vi "split hierarchy.vi"(8 "error in":errorcluster, 10 "UID to split":string, 11 "hierarchy structure":T1) -> (0 "error out":errorcluster, 1 "UIDs moved":string[](array[string]), 2 "hierarchy containing UID":T1, 3 "hierarchy excluding UID":T1)   [LabVIEW 2023, in "CEF.lvlib"]
doc: "Splits a hierarchy at a given instance ID. The first output contains the original tree without the instance specified or any of its children. The second output contains the specified instance and all children, with the specified instance as the new root.Copyright 2017 National Instruments Corporation\n\nLicensed under the Apache License, Version 2.0 (the \"License\"); you may not use this file except in compliance with the License. You may obtain a copy of the License at http://www.apache.org/licenses/LICENSE-2.0\nUnless required by applicable law or agreed to in writing, software distributed under the License is distributed on an \"AS IS\" BASIS, WITHOUT WARRANTIES OR CONDITIONS OF ANY KIND, either express or implied. See the License for the specific language governing permissions and limitations under the License."
uses:
  CEF.lvlib
  hierarchy element.ctl
  hierarchy repo/full hierarchy.ctl
  hierarchy repo/CEF_HierarchyRepo.lvclass
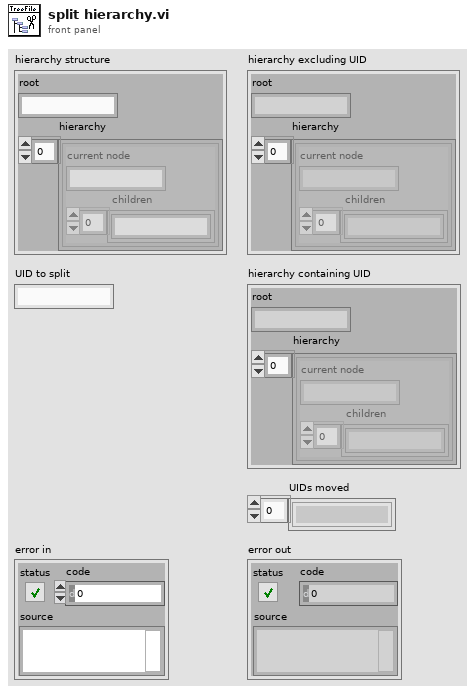
[diagram p1: front panel]
types:
  T1 = typedef "CEF.lvlib/CEF_HierarchyRepo.lvclass/full hierarchy.ctl" = cluster{"root":string, "hierarchy":T2[]}
  T2 = typedef "CEF.lvlib/hierarchy element.ctl" = cluster{"current node":string, "children":string[]}
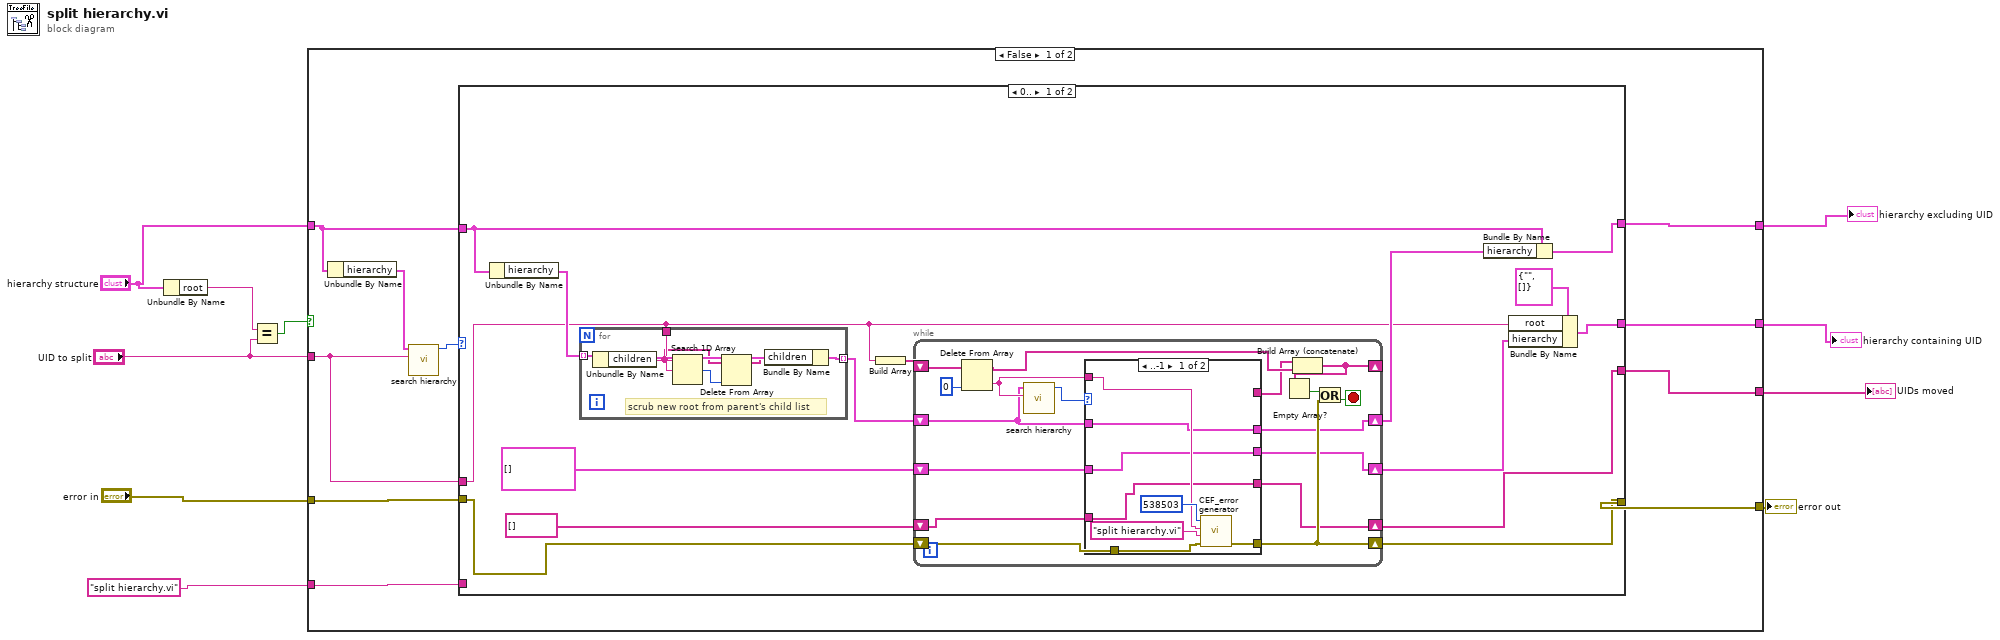
[diagram p0: block diagram]
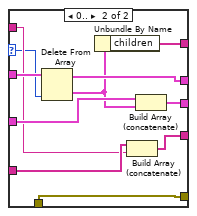
[diagram p2: hidden frame]
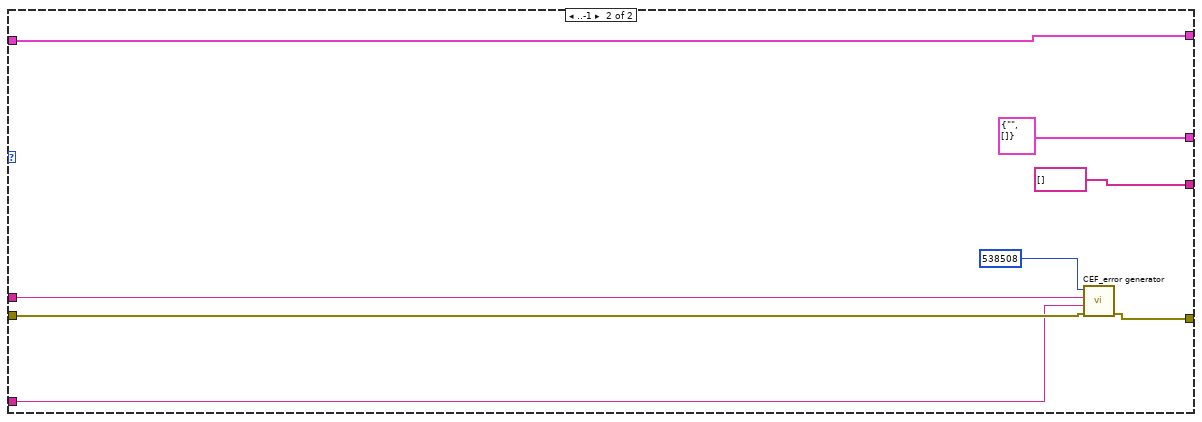
[diagram p3: hidden frame]
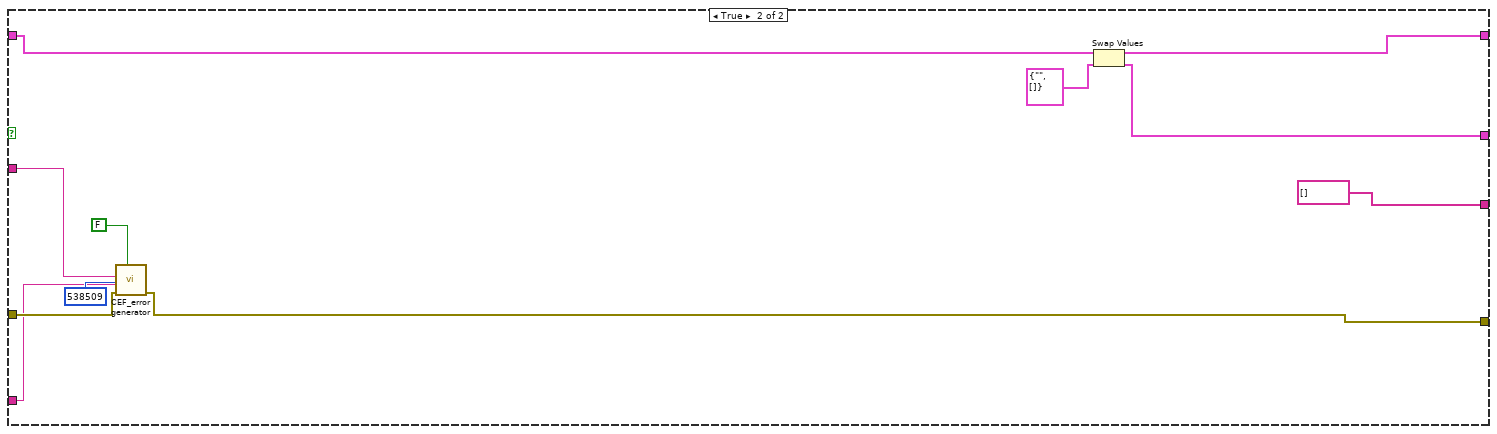
[diagram p4: hidden frame]
diagram:
  n1 = Unbundle By Name("hierarchy structure") -> ("root"=w8:string)
  n2 = Equal?(x=w8, y="UID to split") -> (x = y?=w6:bool)
  n3 = case shown="False" w6 {
    tunnel: "error in" -> [w20 w95]
    tunnel: [w18 w94] -> w9
    tunnel: "UID to split" -> [w17 w93]
    tunnel: [w14 w88] -> w5
    tunnel: "hierarchy structure" -> [w13 w89]
    tunnel: [w11 w86] -> w3
    tunnel: "split hierarchy.vi" ("source") -> [w16 w91]
    tunnel: [w12 string[] [] ("UIDs moved")] -> w1
    frame False {
      n4 = Unbundle By Name(w13) -> ("hierarchy"=w15:T2[])
      n5 = call "search hierarchy.vi"("ID"=w17, "hierarchy"=w15) -> ("index"=w19:i32)  [unwired: 9 in]
      n6 = case shown="0.." w19 {
        tunnel: w20 -> [w25 w84]
        tunnel: [w24 w83] -> w18
        tunnel: w17 -> [w21 w82]
        tunnel: w16 -> [_ w81]
        tunnel: [w33 w80] -> w14
        tunnel: w13 -> [w29 w80]
        tunnel: [w26 string[] [] ("UIDs moved")] -> w12
        tunnel: [w34 T1 {"root"="", "hierarchy"=[]} ("hierarchy structure")] -> w11
        frame 0.. {
          n7 = Unbundle By Name(w29) -> ("hierarchy"=w23:T2[])
          n8 = for {
            tunnel: w23 -> [w41] mode=indexing
            tunnel: [w40] -> w22 mode=indexing
            tunnel: w21 -> [w39]
            # "scrub new root from parent's child list"
            n9 = Unbundle By Name(w41) -> ("children"=w37:string[])
            n10 = Search 1D Array(1D array=w37, element=w39) -> (index of element=w38:i32)  [unwired: 1 in]
            n11 = Delete From Array(array=w37, index=w38) -> (array with subset deleted=w36:string[])  [unwired: 1 in, 1 out]
            n12 = Bundle By Name(cluster=w41, "children"=w36) -> (w40:T2)
          }
          n13 = Build Array(w21) -> (w32:string[])
          n14 = while {
            shift-right: [w42] -> _
            shift-left: w32 -> [w58]
            shift-right: [w46] -> w27
            shift-left: T2[] [] ("hierarchy") -> [w45]
            shift-right: [w48] -> w26
            shift-left: string[] [] ("UIDs moved") -> [w47]
            shift-right: [w50] -> w28
            shift-left: w22 -> [w49]
            shift-right: [w51] -> w24
            shift-left: w25 -> [w53]
            stop <- w56 stop-if-true
            n15 = Delete From Array(array=w58, index=0) -> (deleted portion=w52:string, array with subset deleted=w44:string[])  [unwired: 1 in]
            n16 = call "search hierarchy.vi"("ID"=w52, "hierarchy"=w49) -> ("index"=w54:i32)  [unwired: 9 in]
            n17 = case shown="..-1" w54 {
              selector: w54 -> [_ w67]
              tunnel: [w64 w77] -> w51
              tunnel: w53 -> [w63 w77]
              tunnel: w52 -> [w62 w70]
              tunnel: [w61 w75] -> w50
              tunnel: w49 -> [w61 w76]
              tunnel: [w60 w73] -> w48
              tunnel: w47 -> [w60 w74]
              tunnel: [w59 w71] -> w46
              tunnel: w45 -> [w59 w72]
              tunnel: [_ w68] -> w43
              frame ..-1 {
                n18 = call "CEF_error generator.vi"("error in"=w63, "source"="split hierarchy.vi", "append error message"=w62, "error code (0)"=538503) -> ("error out"=w64:errorcluster)  [unwired: 5 in]
              }
              frame 0.. {
                n19 = Delete From Array(array=w76, index=w67) -> (deleted portion=w69:T2, array with subset deleted=w75:T2[])  [unwired: 1 in]
                n20 = Unbundle By Name(w69) -> ("children"=w68:string[])
                n21 = Build Array (concatenate)(w74, w70) -> (w73:string[])
                n22 = Build Array (concatenate)(w72, w69) -> (w71:T2[])
              }
            }
            n23 = Build Array (concatenate)(w43, w44) -> (w42:string[])
            n24 = Empty Array?(array=w42) -> (empty?=w55:bool)
            n25 = Or(x=w55, y=w51) -> (x .or. y?=w56:bool)
          }
          n26 = Bundle By Name(cluster=w29, "hierarchy"=w28) -> (w33:T1)
          n27 = Bundle By Name(cluster=T1 {"root"="", "hierarchy"=[]} ("hierarchy structure"), "root"=w21, "hierarchy"=w27) -> (w34:T1)
        }
        frame ..-1 {
          n28 = call "CEF_error generator.vi"("error in"=w84, "source"=w81, "append error message"=w82, "error code (0)"=538508) -> ("error out"=w83:errorcluster)  [unwired: 5 in]
        }
      }
    }
    frame True {
      n29 = call "CEF_error generator.vi"("error (T)"=FALSE, "error in"=w95, "source"=w91, "append error message"=w93, "error code (0)"=538509) -> ("error out"=w94:errorcluster)  [unwired: 4 in]
      n30 = Swap Values(12:w89, 14:T1 {"root"="", "hierarchy"=[]} ("y'")) -> (1:w88:T1, 3:w86:T1)  [unwired: 1 in]
    }
  }
  "error out" <- w9
  "hierarchy excluding UID" <- w5
  "hierarchy containing UID" <- w3
  "UIDs moved" <- w1
